vi "verify expouse time.vi"(8 "error in (no error)":errorcluster, 11 "Simulated_CCD_Camera in":refnum<class "Simulated_CCD_Camera.lvclass">) -> (0 "error out":errorcluster, 3 "Simulated_CCD_Camera out":refnum<class "Simulated_CCD_Camera.lvclass">)   [LabVIEW 2018, in "Simulated_CCD_Camera.lvclass"]
uses:
  Simulated_CCD_Camera.lvclass
  Simulated_CCD_Camera.lvclass/Simulated_CCD_Camera.ctl
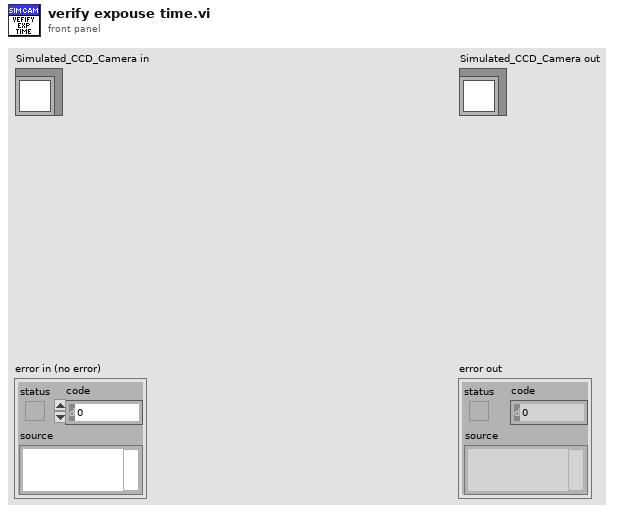
[diagram p1: front panel]
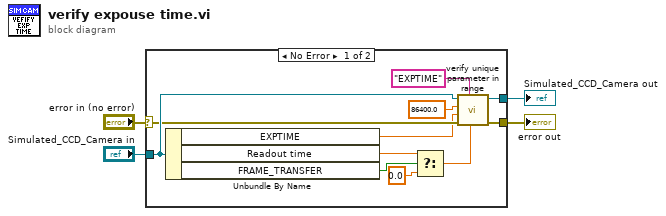
[diagram p0: block diagram]
diagram:
  n1 = case shown="No Error" "error in (no error)" {
    selector: "error in (no error)" -> [w12 w17]
    tunnel: [w15 w17] -> w3
    tunnel: [w14 w16] -> w1
    tunnel: "Simulated_CCD_Camera in" -> [w13 w16]
    frame No Error {
      n2 = Unbundle By Name(w13) -> ("EXPTIME"=w11:dbl, "Readout time"=w8:dbl, "FRAME_TRANSFER"=w9:bool)
      n3 = Select(t=w8, s=w9, f=0.0) -> (s? t:f=w7:dbl)
      n4 = call "verify unique parameter in range.vi"("lower limit"=w7, "parameter name"="EXPTIME", "error in (no error)"=w12, "value"=w11, "upper limit"=86400.0, "Simulated_CCD_Camera in"=w13) -> ("error out"=w15:errorcluster, "Simulated_CCD_Camera out"=w14:refnum<class "Simulated_CCD_Camera.lvclass">)  [unwired: 4 in]
    }
    frame Error {
    }
  }
  "error out" <- w3
  "Simulated_CCD_Camera out" <- w1
